vi "Enqueue.vi"(8 "错误输入（无错误）":errorcluster, 9 "Steps":T1[](array[typedef]), 10 "Comd":enum16{"Top", "Bottom", "Nothing"}(ring), 11 "队列输入":refnum<queue>) -> (0 "error out":errorcluster, 3 "队列输出":refnum<queue>)   [LabVIEW 2016]
uses:
  Ctls/Auto Steps.ctl
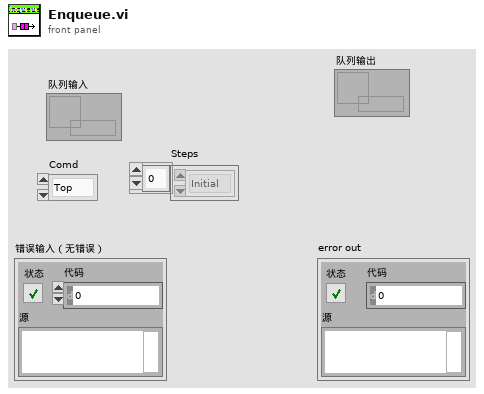
[diagram p1: front panel]
types:
  T1 = typedef "Auto Steps.ctl" = enum16{"Nothing", "Initial", "ReadConf", "WaitTrigger", "SnapOnce", "Rotate180", "SnapSecond", "SendPos", "Error", "Pause", "Exit"}
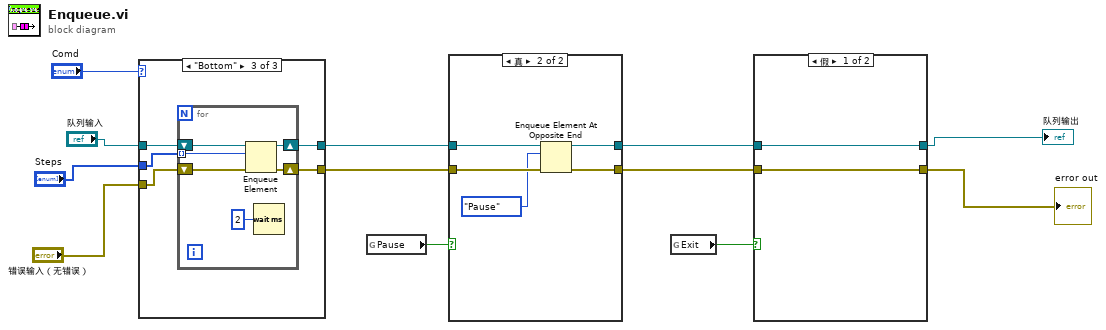
[diagram p0: block diagram]
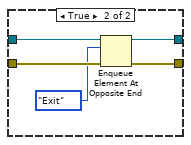
[diagram p2: hidden frame]
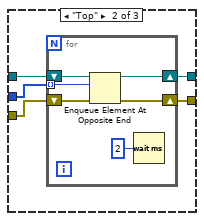
[diagram p5: hidden frame]
diagram:
  n1 = case shown="\"Bottom\"" "Comd" {
    tunnel: "队列输入" -> [w14 w16 w30]
    tunnel: [w14 w17 w29] -> w8
    tunnel: "错误输入（无错误）" -> [w13 w19 w28]
    tunnel: [w13 w18 w27] -> w7
    tunnel: "Steps" -> [_ w15 w26]
    frame "Nothing", Default {
    }
    frame "Top" {
      n2 = for {
        tunnel: w15 -> [w21] mode=indexing
        shift-right: [w24] -> w18
        shift-left: w19 -> [w25]
        shift-right: [w23] -> w17
        shift-left: w16 -> [w22]
        n3 = Enqueue Element At Opposite End(queue=w22, element=w21, error in (no error)=w25) -> (queue out=w23:refnum<queue>, error out=w24:errorcluster)  [unwired: 1 in, 1 out]
        n4 = Wait (ms)(milliseconds to wait=u32 2 ("等待时间（毫秒）")) -> ()  [unwired: 1 out]
      }
    }
    frame "Bottom" {
      n5 = for {
        tunnel: w26 -> [w32] mode=indexing
        shift-right: [w35] -> w29
        shift-left: w30 -> [w36]
        shift-right: [w33] -> w27
        shift-left: w28 -> [w34]
        n6 = Enqueue Element(queue=w36, element=w32, error in (no error)=w34) -> (queue out=w35:refnum<queue>, error out=w33:errorcluster)  [unwired: 1 in, 1 out]
        n7 = Wait (ms)(milliseconds to wait=u32 2 ("等待时间（毫秒）")) -> ()  [unwired: 1 out]
      }
    }
  }
  n8 = global read "全局 1.vi" "Pause"() -> (w9:bool)
  n9 = case shown="真" w9 {
    tunnel: w8 -> [w38 w43]
    tunnel: w7 -> [w37 w42]
    tunnel: [w38 w40] -> w6
    tunnel: [w37 w39] -> w5
    frame False {
    }
    frame True {
      n10 = Enqueue Element At Opposite End(queue=w43, element=Auto_Steps."Pause" ("Steps 2"), error in (no error)=w42) -> (queue out=w40:refnum<queue>, error out=w39:errorcluster)  [unwired: 1 in, 1 out]
    }
  }
  n11 = global read "全局 1.vi" "Exit"() -> (w4:bool)
  n12 = case shown="假" w4 {
    tunnel: w6 -> [w45 w50]
    tunnel: w5 -> [w44 w49]
    tunnel: [w45 w47] -> w3
    tunnel: [w44 w46] -> w2
    frame False {
    }
    frame True {
      n13 = Enqueue Element At Opposite End(queue=w50, element=Auto_Steps."Exit" ("Steps 2"), error in (no error)=w49) -> (queue out=w47:refnum<queue>, error out=w46:errorcluster)  [unwired: 1 in, 1 out]
    }
  }
  "队列输出" <- w3
  "error out" <- w2
